vi "GE 5565PIORC.Registers.NIC.Network Interrupt Command.Get.vi"(8 "error in (no error)":errorcluster, 11 "GE 5565PIORC in":refnum<class "GE 5565PIORC.lvclass">) -> (0 "error out":errorcluster, 2 "Network Interrupt Command":u8, 3 "GE 5565PIORC out":refnum<class "GE 5565PIORC.lvclass">)   [LabVIEW 2016, in "GE 5565PIORC.lvclass"]
doc: "An 8-bit register containing a four-bit code that defines the type of network interrupt issued. See Table 3-49 for a definition of the possible codes. The NIC is both read and write accessible. Only writing to the NIC register will initiate the network interrupt. The network interrupt is transmitted in order following after all previously written data.\n\n<B>NIC[3,2,1,0]</B> - <B>Function</B>\nX000 - Reset Node Request\nX001 - Network Interrupt 1 (stored in a 127 deep FIFO at the receiving node)\nX010 - Network Interrupt 2 (stored in a 127 deep FIFO at the receiving node)\nX011 - Network Interrupt 3 (stored in a 127 deep FIFO at the receiving node)\nX100 - Reserved (Setting to this type will only set the OWN DATA bit in the LCSR1)\nX101 - Reserved (Setting to this type will only set the OWN DATA bit in the LCSR1)\nX110 - Reserved (Setting to this type will only set the OWN DATA bit in the LCSR1)\nX111 - Network Interrupt 4 (stored in a 127 deep FIFO at the receiving node)\n1XXX - Global enable. Send to all nodes regardless of NTN Register"
uses:
  GE 5565PIORC.lvclass
  GE 5565PIORC.Registers.RFM Control and Status.ctl
  GE 5565PIORC.lvclass/GE 5565PIORC.ctl
  GE 5565PIORC.Register.RFM Control and Status.Read (U8).vi
  GE 5565PIORC.Register.Read.vi
  GE 5565PIORC.Register.Read (U8).vi
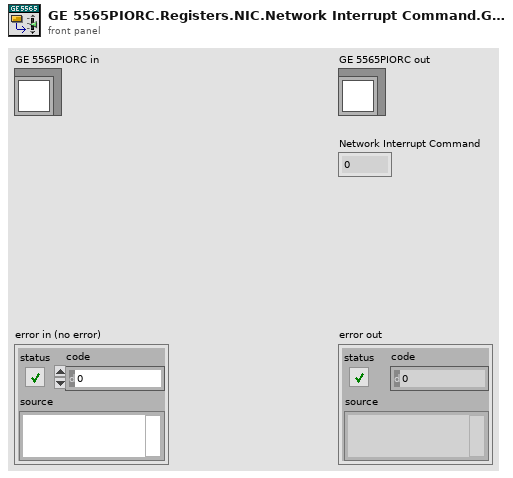
[diagram p1: front panel]
types:
  T1 = typedef "GE 5565PIORC.lvclass/GE 5565PIORC.Registers.RFM Control and Status.ctl" = u32
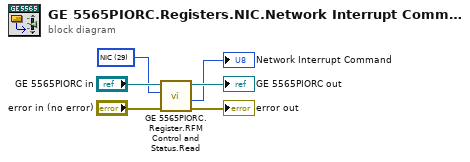
[diagram p0: block diagram]
diagram:
  w1 = T1 29 items=["BRV"=0, "BID"=1, "BRB"=2, "NID"=4, "LCSR1"=8, "LISR"=16, "LIER"=20, "NTD"=24, "NTN"=28, "NIC"=29, "ISD1"=32, "SID1"=36, "ISD2"=40, "SID2"=44, "ISD3"=48, "SID3"=52, "ISD4"=56, "SID4"=60] ("Register")
  n1 = call-poly "GE 5565PIORC.Register.RFM Control and Status.Read.vi"("error in (no error)"="error in (no error)", "Register"=w1, "GE 5565PIORC in"="GE 5565PIORC in") -> ("error out"=→"error out":errorcluster, "Value"=→"Network Interrupt Command":u8, "GE 5565PIORC out"=→"GE 5565PIORC out":refnum<class "GE 5565PIORC.lvclass">)  [unwired: 6 in]
